vi "Global 4.vi"() -> ()   [LabVIEW 2024]
panel:
  in  "x":dbl
  in  "y":dbl
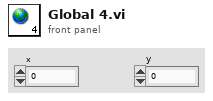
[diagram p1: front panel]
diagram:
